vi "time date filename.vi"(7 "file name in":string="fred") -> (8 "time date file name out":string)   [LabVIEW 2019]
doc: "this subvi adds a time date stamp to a file name for uniqueness\n\nPaul K Dixon\nP350\nCSUSB Physics"
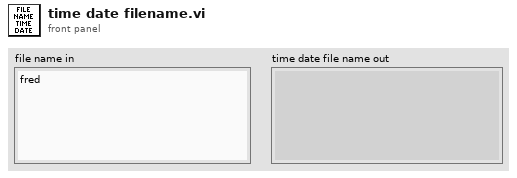
[diagram p1: front panel]
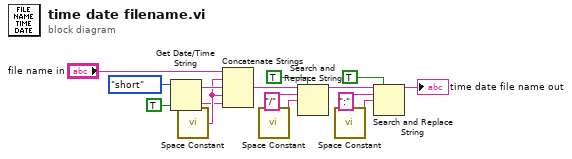
[diagram p0: block diagram]
diagram:
  n1 = Get Date/Time String(date format (0)=enum16{"short", "long", "abbreviated"}."short", want seconds? (F)=TRUE) -> (date string=w12:string, time string=w6:string)  [unwired: 1 in]
  n2 = call <vilib>:"Space Constant.vi"() -> ("String"=w7:string)
  n3 = Concatenate Strings("file name in", w7, w12, w7, w6) -> (w11:string)
  n4 = call <vilib>:"Space Constant.vi"() -> ("String"=w9:string)
  n5 = Search and Replace String(replace all?=TRUE ("replace all? (F)"), input string=w11, search string="/", replace string=w9) -> (result string=w2:string)  [unwired: 4 in, 3 out]
  n6 = call <vilib>:"Space Constant.vi"() -> ("String"=w4:string)
  n7 = Search and Replace String(replace all?=TRUE ("replace all? (F)"), input string=w2, search string=":", replace string=w4) -> (result string=→"time date file name out":string)  [unwired: 4 in, 3 out]
